vi "MeasureRMS.vi"(9 "error in":errorcluster, 10 "Number of Samples":i32=1000, 11 "Rate":dbl=100000.0) -> (0 "error out":errorcluster, 1 "RMS Voltage":dbl format="%0.2f", 2 "Waveform Graph":dynamicdata(graph))   [LabVIEW 2014]
doc: "Measures the analog signal and gives out the rms value and a waveform for the given signal. The VI takes a sampling rate and number of samples."
uses:
  <vilib>/Analysis/NI_AALPro.lvlib
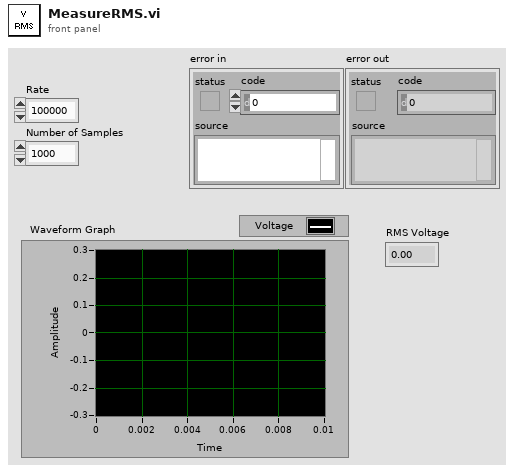
[diagram p1: front panel]
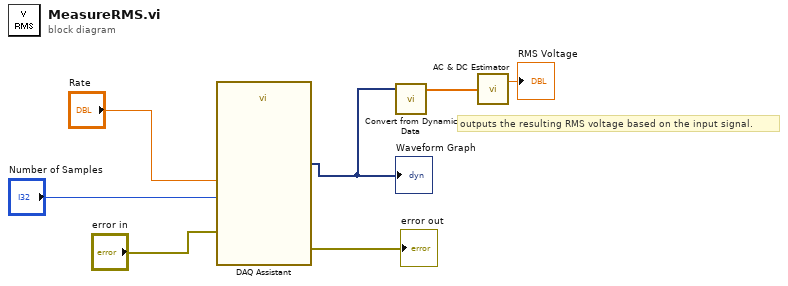
[diagram p0: block diagram]
diagram:
  # "outputs the resulting RMS voltage based on the input signal."
  n1 = call "DAQ Assistant"("rate"="Rate", "number of samples"="Number of Samples", "error in"="error in") -> ("data"=w3:dynamicdata, "error out"=→"error out":errorcluster)  [unwired: 14 in, 1 out]
  "Waveform Graph" <- w3
  n2 = call "Convert from Dynamic Data"("Dynamic Data Type"=w3) -> ("Array"=w2:dbl[])  [unwired: 3 in]
  n3 = call <vilib>:"AC & DC Estimator.vi"("Signal (V)"=w2) -> ("AC estimate (Vrms)"=→"RMS Voltage":dbl)  [unwired: 1 out]
